vi "rtree query callback.vi"(7 "pContext":u32, 8 "error in (no error)":errorcluster, 9 "?":i32, 10 "zQueryFunc":string, 11 "db":dbl) -> (0 "error out":errorcluster, 2 "function return":i32, 3 "db out":dbl, 5 "pContext out":u32)   [LabVIEW 2020, in "sqlite3.lvlib"]
uses:
  sqlite3.lvlib
  errstr.vi
  bin/sqlite3_64.dll
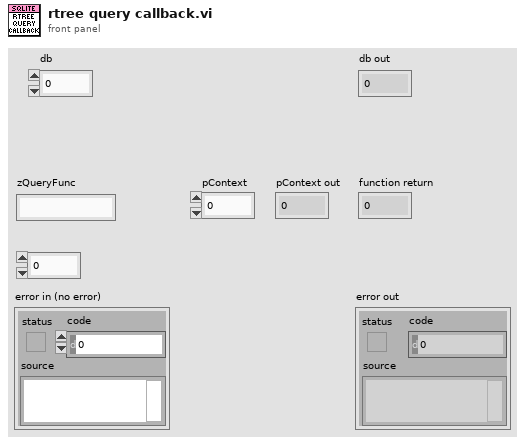
[diagram p1: front panel]
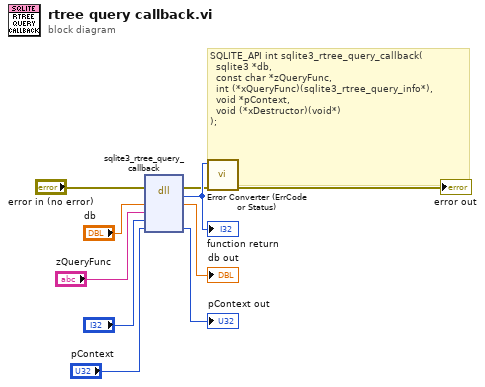
[diagram p0: block diagram]
diagram:
  # "SQLITE_API int sqlite3_rtree_query_callback(\n  sqlite3 *db,\n  const char *zQueryFunc,\n  int (*xQueryFunc)(sqlite3_rtree_query_info*),\n  void *pContext,\n  void (*xDestructor)(void*)\n);"
  n1 = dll-call lib="C:/Users/Fred.Guo/Desktop/Database-configuration/externals/sqlite3/Source/bin/sqlite3_*.*" fn="sqlite3_rtree_query_callback"(error in="error in (no error)", "db"="db", "zQueryFunc"="zQueryFunc", "?", "pContext"="pContext") -> (error out=w2:errorcluster, w10:i32, "db"=→"db out":dbl, "pContext"=→"pContext out":u32)  [unwired: 4 in, 1 out]
  "function return" <- w10
  n2 = call "Error Converter (ErrCode or Status).vi"("error in (no error)"=w2, "error code"=w10) -> ("error out"=→"error out":errorcluster)  [unwired: 9 in]
